vi "myRIO_Brig_RT__Case_Exp_State_initBlock__v2.vi"(1 "input_spout":enum16{"Left", "Right"}(ring), 7 "input_dataCurrent":u16[](array[numeric]), 9 "input_dataExp":u16[](array[numeric]), 11 "input_dataBlock":u16[][](array[numeric])) -> (2 "output_state":T1=enum."initTrial", 3 "output_spout":enum16{"Left", "Right"}(ring), 4 "idxDataBlock":i32, 8 "output_dataCurrent":u16[](array[numeric]), 10 "output_dataExp":u16[](array[numeric]), 13 "output_TpB_target":u16, 14 "output_iBlock":u16, 15 "output_dataBlock":u16[][](array[numeric]))   [LabVIEW 2014]
uses:
  myRIO_BRig_RT__Case_Exp_stateList.ctl
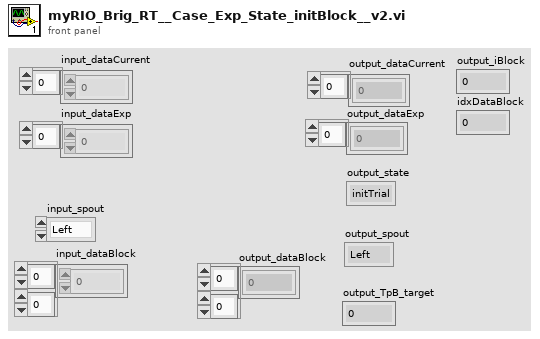
[diagram p1: front panel]
types:
  T1 = typedef "myRIO_BRig_RT__Case_Exp_stateList.ctl" = enum16{"Start1", "Start2", "Start3", "saveSettings1", "saveSettings2", "saveSettings3", "saveSettings4", "saveSettings_LC_ENL_l1", "saveSettings_LC_ENL_l2", "saveSettings_LC_Cue_l1", "saveSettings_LC_Cue_l2", "saveSettings6_LC_l1_Other", "SaveSettings6_LC_l2_Other", "setSettings_Audio", "setSettings_Laser", "initBlock_pre", "initBlock", "initBlock2", "initBlock_post", "initTrial_pre", "initTrial", "initTrial2", "initTrial3", "initTrial4", "initTrial_LC_ENL1", "initTrial_LC_Cue1", "initTrial_LC_Cue1_2", "initTrial_LC_Sel", "initTrial_post", "ENL1_pre", "ENL1", "ENL1_post", "ENL1Penalty_pre", "ENL1Penalty", "ENL2_pre", "ENL2", "ENL2Penalty_pre", "ENL2Penalty", "Cue1_pre", "Cue1", "Cue1_post", "Cue1Penalty_pre", "Cue1Penalty", "Cue2_pre", "Cue2", "Cue2Penalty_pre", "Cue2Penalty", "Selection_pre", "Selection", "Select_post", "SelectReward_pre", "SelectReward", "SelectRewardPost_pre", "SelectRewardPost", "SelectWrong_pre", "SelectWrong", "SelectWrong_post", "SelectTimeout_pre", "SelectTimeout", "SelectTimeout_post", "endTrial_pre", "endTrial1", "endTrial2", "endTrial3", "endTrial_post", "endBlock_pre", "endBlock", "endBlock_post", "endExp", "commConnect", "commUpload_pre", "commUpload_dataBlock", "commUpload_dataCurrent", "commUpload_dataExp", "commUpload_dataLC", "commUpload_dataTrial", "commUpload_post", "saveData_pre", "saveData_dataBlock", "saveData_dataCurrent", "saveData_dataExp", "saveData_dataLC", "saveData_dataTrial", "saveData_post", "empty_endBlock1", "empty_endBlock2", "empty_endTrial1", "empty_endTrial2", "empty_endTrial3", "empty_endTrial4", "empty_endTrial5", "dummyState", "dummyState_endBlock"}
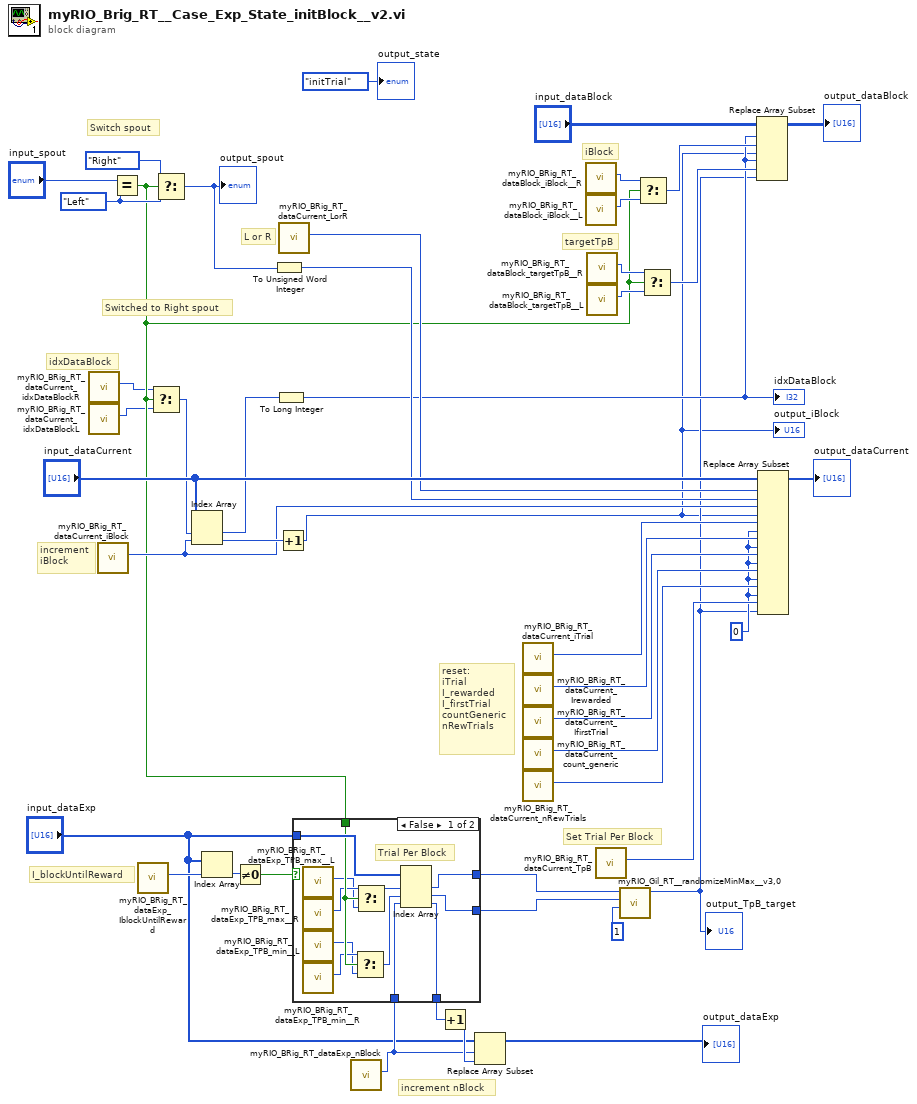
[diagram p0: block diagram]
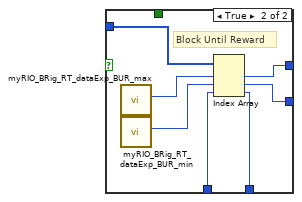
[diagram p2: hidden frame]
diagram:
  w14 = u16 0
  w45 = enum16{"Left", "Right"}."Left"
  # "idxDataBlock"
  # "Switched to Right spout"
  # "targetTpB"
  # "iBlock"
  # "L or R"
  # "I_blockUntilReward"
  # "increment nBlock"
  # "reset:\niTrial\nI_rewarded\nI_firstTrial\ncountGeneric\nnRewTrials"
  # "increment\niBlock"
  # "Set Trial Per Block"
  # "Switch spout"
  n1 = call "myRIO_BRig_RT_dataCurrent_idxDataBlockR.vi"() -> ("output_idxDataBlock__R"=w7:i32)  [unwired: 11 in]
  n2 = call "myRIO_BRig_RT_dataCurrent_idxDataBlockL.vi"() -> ("output_idxDataBlock__L"=w6:i32)  [unwired: 11 in]
  n3 = call "myRIO_BRig_RT_dataCurrent_iBlock.vi"() -> ("output_iBlock"=w9:i32)  [unwired: 11 in]
  n4 = Equal?(x="input_spout", y=w45) -> (x = y?=w8:bool)
  n5 = call "myRIO_BRig_RT_dataExp_IblockUntilReward.vi"() -> ("output_I_blockUntilReward"=w30:i32)  [unwired: 11 in]
  n6 = Select(t=w7, s=w8, f=w6) -> (s? t:f=w5:i32)
  n7 = Select(t=enum16{"Left", "Right"}."Right", s=w8, f=w45) -> (s? t:f=w23:enum16{"Left", "Right"})
  "output_spout" <- w23
  n8 = Index Array(array="input_dataCurrent", index #1=w5, index #2=w9) -> (element #1=w4:u16, element #2=w40:u16)
  n9 = Index Array(array="input_dataExp", index=w30) -> (element=w29:u16)
  n10 = Not Equal To 0?(x=w29) -> (x != 0?=w28:bool)
  n11 = To Unsigned Word Integer(number=w23) -> (unsigned 16bit integer=w17:u16)
  n12 = To Long Integer(number=w4) -> (32bit integer=w3:i32)
  "idxDataBlock" <- w3
  n13 = Increment(x=w40) -> (x+1=w1:u16)
  "output_iBlock" <- w1
  n14 = call "myRIO_BRig_RT_dataCurrent_LorR.vi"() -> ("output_LorR"=w18:i32)  [unwired: 11 in]
  n15 = call "myRIO_BRig_RT_dataExp_nBlock.vi"() -> ("output_nBlock"=w34:i32)  [unwired: 11 in]
  n16 = case shown="False" w28 {
    tunnel: w34 -> [w55 w62]
    tunnel: [w54 w61] -> w33
    tunnel: "input_dataExp" -> [w57 w60]
    tunnel: [w52 w59] -> w26
    tunnel: [w53 w58] -> w25
    tunnel: w8 -> [w56 _]
    frame False {
      # "Trial Per Block"
      n17 = call "myRIO_BRig_RT_dataExp_TPB_max__L.vi"() -> ("output_TPB_max__L"=w46:i32)  [unwired: 11 in]
      n18 = call "myRIO_BRig_RT_dataExp_TPB_max__R.vi"() -> ("output_TPB_max__R"=w47:i32)  [unwired: 11 in]
      n19 = call "myRIO_BRig_RT_dataExp_TPB_min__L.vi"() -> ("output_TPB_min__L"=w48:i32)  [unwired: 11 in]
      n20 = call "myRIO_BRig_RT_dataExp_TPB_min__R.vi"() -> ("output_TPB_min__R"=w49:i32)  [unwired: 11 in]
      n21 = Select(t=w49, s=w56, f=w48) -> (s? t:f=w50:i32)
      n22 = Select(t=w47, s=w56, f=w46) -> (s? t:f=w51:i32)
      n23 = Index Array(array=w57, index #1=w51, index #2=w50, index #3=w55) -> (element #1=w52:u16, element #2=w53:u16, element #3=w54:u16)
    }
    frame True {
      # "Block Until Reward"
      n24 = call "myRIO_BRig_RT_dataExp_BUR_max.vi"() -> ("output_BUR_max"=w64:i32)  [unwired: 11 in]
      n25 = call "myRIO_BRig_RT_dataExp_BUR_min.vi"() -> ("output_BUR_min"=w63:i32)  [unwired: 11 in]
      n26 = Index Array(array=w60, index #1=w64, index #2=w63, index #3=w62) -> (element #1=w59:u16, element #2=w58:u16, element #3=w61:u16)
    }
  }
  n27 = Increment(x=w33) -> (x+1=w36:u16)
  n28 = Replace Array Subset(array="input_dataExp", new element=w36, index=w34) -> (→"output_dataExp":u16[])
  n29 = call "myRIO_BRig_RT_dataCurrent_iTrial.vi"() -> ("output_iTrial"=w39:i32)  [unwired: 11 in]
  n30 = call "myRIO_BRig_RT_dataCurrent_Irewarded.vi"() -> ("output_I_rewarded"=w38:i32)  [unwired: 11 in]
  n31 = call "myRIO_BRig_RT_dataCurrent_IfirstTrial.vi"() -> ("output_I_firstTrial"=w37:i32)  [unwired: 11 in]
  n32 = call "myRIO_BRig_RT_dataCurrent_count_generic.vi"() -> ("output_count_generic"=w31:i32)  [unwired: 11 in]
  n33 = call "myRIO_BRig_RT_dataCurrent_nRewTrials.vi"() -> ("output_nRewTrials"=w15:i32)  [unwired: 11 in]
  n34 = call "myRIO_BRig_RT_dataBlock_iBlock__R.vi"() -> ("output_iBlock__R"=w13:i32)  [unwired: 11 in]
  n35 = call "myRIO_BRig_RT_dataBlock_iBlock__L.vi"() -> ("output_iBlock__L"=w12:i32)  [unwired: 11 in]
  n36 = call "myRIO_BRig_RT_dataBlock_targetTpB__R.vi"() -> ("output_targetTpB__R"=w11:i32)  [unwired: 11 in]
  n37 = call "myRIO_BRig_RT_dataBlock_targetTpB__L.vi"() -> ("output_targetTpB__L"=w10:i32)  [unwired: 11 in]
  n38 = call "myRIO_BRig_RT_dataCurrent_TpB.vi"() -> ("output_TpB"=w16:i32)  [unwired: 11 in]
  n39 = call "myRIO_Gil_RT__randomizeMinMax__v3,0.vi"("Input_Increment"=u16 1, "Input_Min"=w25, "Input_Max"=w26) -> ("Output"=w2:u16)  [unwired: 8 in]
  "output_TpB_target" <- w2
  n40 = Select(t=w13, s=w8, f=w12) -> (s? t:f=w21:i32)
  n41 = Select(t=w11, s=w8, f=w10) -> (s? t:f=w20:i32)
  n42 = Replace Array Subset(array="input_dataBlock", new element #1=w1, index (row) #1=w3, index (col) #1=w21, new element #2=w2, index (row) #2=w3, index (col) #2=w20) -> (→"output_dataBlock":u16[][])
  n43 = Replace Array Subset(array="input_dataCurrent", new element #1=w17, index #1=w18, new element #2=w1, index #2=w9, new element #3=w14, index #3=w39, new element #4=w14, index #4=w38, new element #5=w14, index #5=w37, new element #6=w14, index #6=w31, new element #7=w14, index #7=w15, new element #8=w2, index #8=w16) -> (→"output_dataCurrent":u16[])
  "output_state" <- myRIO_BRig_RT__Case_Exp_stateList."initTrial" ("Enum")
